vi "Collector.vi"(6 "MotorSpeed":dbl, 7 "Action":T10, 8 "Error in":errorcluster, 9 "BottomLS":T8={"DevStatus"={"status"=FALSE, "code"=0, "source"=""}, "DIO Channel"=enum."Invalid", "Digital Module"=enum."Digital Module 1"}, 10 "TopLS":T8={"DevStatus"={"status"=FALSE, "code"=0, "source"=""}, "DIO Channel"=enum."Invalid", "Digital Module"=enum."Digital Module 1"}, 11 "Motor":T1={"DeviceStatus"={"status"=FALSE, "code"=0, "source"=""}, "Type"=enum."PWM", "PWM"={"Digital Module"=enum."Digital Module 1", "PWM Channel"=enum."Invalid", "DeadBand"={"Name"="", "maxPositivePwm"=0, "minPositivePwm"=0, "centerPwm"=0, "maxNegativePwm"=0, "minNegativePwm"=0, "angularRange"=0}}, "CAN"={"Device Number"=0, "Control Mode"=enum."Percent VBus", "Semaphore"=refnum, "Max Vout"=12.0}, "Invert"=FALSE, "TransformRef"=refnum, "InvTransformRef"=refnum}) -> (0 "Error out":errorcluster, 1 "Lower Triggered?":bool, 2 "Upper Triggered?":bool)   [LabVIEW 2013]
doc: "Controls the collector arm, along with the two sets of limit switches associated with it (one set all the way up, the other all the way down). NOTE: all states return the status of the limit switches. It has the following actions:\n-Init: takes references to the motor and limit switches and stores them in shift registers\n-Raise: attempts to raise the collector (nothing happens if the upper limit switch is triggered)\n-Lower: attempts to lower the collector (nothing happens if the lower limit switch is triggered)\n-Stop: stops the motor\n-GetStatus: returns the value of the limit switches"
uses:
  CollectorAction.ctl
  <vilib>/Rock Robotics/WPI/DigitalInput/WPI_DigitalInputDevRef.ctl
  <vilib>/Rock Robotics/SystemInterfaces/DIO/FPGA_DIOChannel.ctl
  <vilib>/Rock Robotics/SystemInterfaces/Typedef/FPGA_TypedefDigitalModule.ctl
  <vilib>/Rock Robotics/WPI/MotorControl/WPI_MotorControlDeviceRef.ctl
  <vilib>/Rock Robotics/SystemInterfaces/DIO/FPGA_DIOPWMChannel.ctl
  <vilib>/Rock Robotics/WPI/PWM/WPI_PWMDeadband.ctl
  <vilib>/Rock Robotics/WPI/CAN/Jaguar/SubVIs/WPI_CANJaguar_ControlMode.ctl
  <vilib>/Rock Robotics/WPI/PWM/WPI_PWMTransform_ConPane.ctl
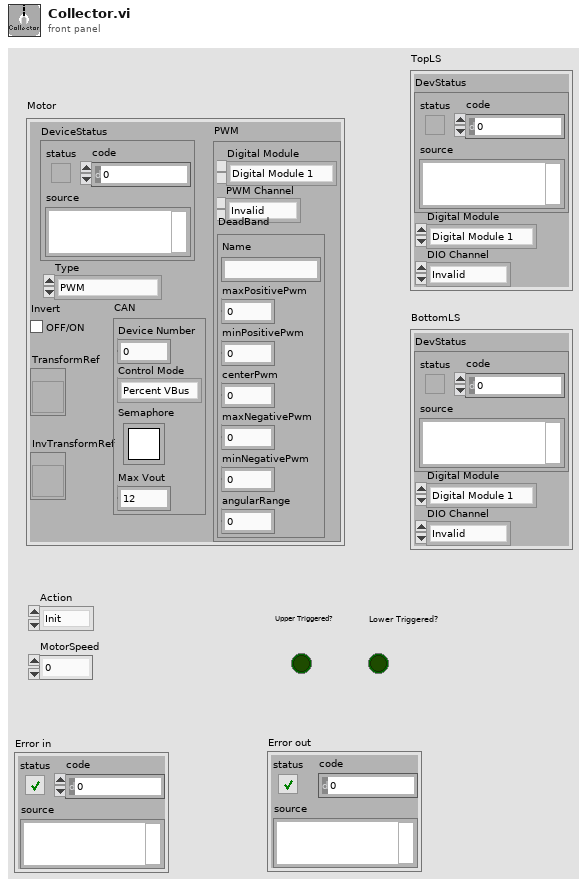
[diagram p1: front panel]
types:
  T1 = typedef "WPI_MotorControlDeviceRef.ctl" = cluster{"DeviceStatus":errorcluster, "Type":enum16{"PWM", "CAN"}, "PWM":cluster{"Digital Module":T2, "PWM Channel":T3, "DeadBand":T4}, "CAN":cluster{"Device Number":u8, "Control Mode":T5, "Semaphore":T6, "Max Vout":dbl}, "Invert":bool, "TransformRef":T7, "InvTransformRef":T7}
  T2 = typedef "FPGA_TypedefDigitalModule.ctl" = enum16{"Digital Module 1", "Digital Module 2"}
  T3 = typedef "FPGA_DIOPWMChannel.ctl" = enum8{"PWM 1", "PWM 2", "PWM 3", "PWM 4", "PWM 5", "PWM 6", "PWM 7", "PWM 8", "PWM 9", "PWM 10", "Invalid"}
  T4 = typedef "WPI_PWMDeadband.ctl" = cluster{"Name":string, "maxPositivePwm":i32, "minPositivePwm":i32, "centerPwm":i32, "maxNegativePwm":i32, "minNegativePwm":i32, "angularRange":u16}
  T5 = typedef "WPI_CANJaguar_ControlMode.ctl" = enum8{"Percent VBus", "Current", "Speed", "Position", "Voltage"}
  T6 = typedef "Semaphore RefNum" = refnum<k1>
  T7 = typedef "WPI_PWMTransform_ConPane.ctl" = refnum<vi>
  T8 = typedef "WPI_DigitalInputDevRef.ctl" = cluster{"DevStatus":errorcluster, "DIO Channel":T9, "Digital Module":T2}
  T9 = typedef "FPGA_DIOChannel.ctl" = enum8{"DIO 1", "DIO 2", "DIO 3", "DIO 4", "DIO 5", "DIO 6", "DIO 7", "DIO 8", "DIO 9", "DIO 10", "DIO 11", "DIO 12", "DIO 13", "DIO 14", "Invalid"}
  T10 = typedef "CollectorAction.ctl" = enum16{"Init", "Raise", "Lower", "Stop", "GetStatus"}
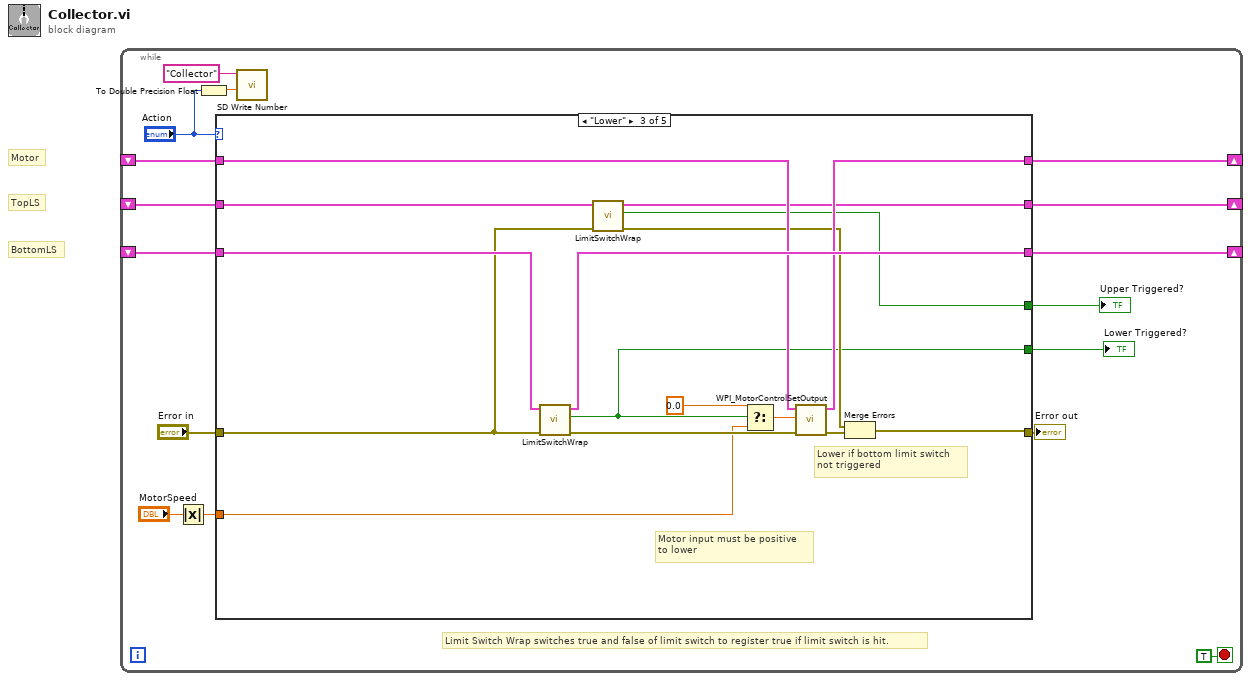
[diagram p0: block diagram]
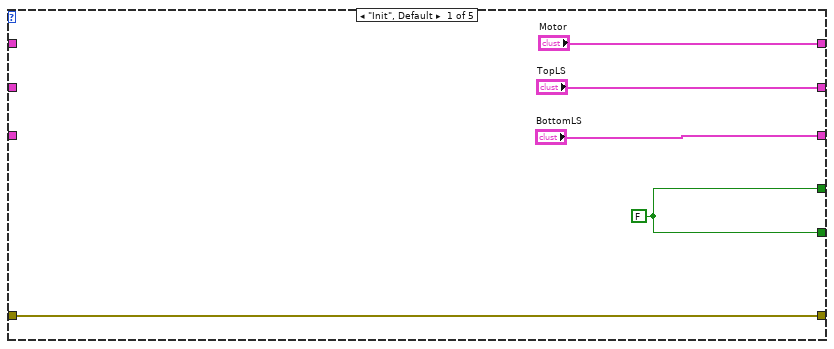
[diagram p2: hidden frame]
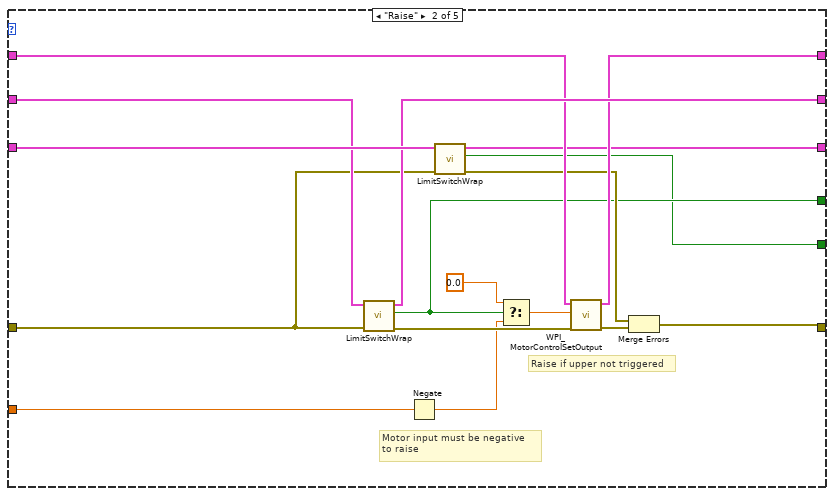
[diagram p3: hidden frame]
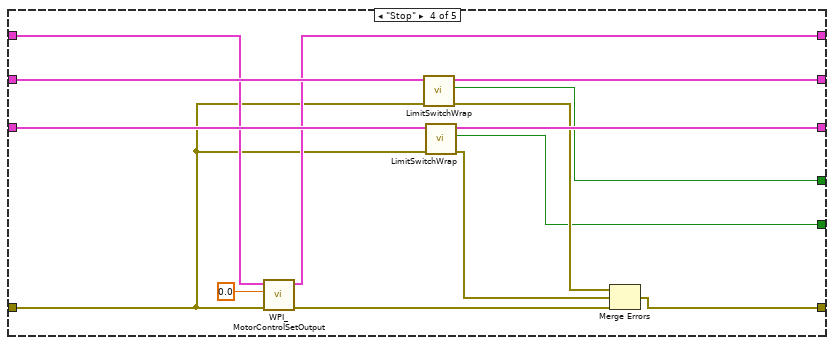
[diagram p4: hidden frame]
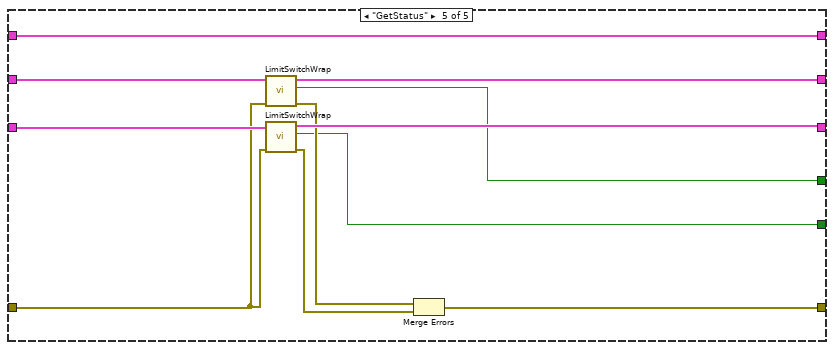
[diagram p5: hidden frame]
diagram:
  # "BottomLS"
  # "TopLS"
  # "Motor"
  n1 = while {
    shift-right: [w13] -> _
    shift-left: _ -> [w10]
    shift-right: [w14] -> _
    shift-left: _ -> [w11]
    shift-right: [w15] -> _
    shift-left: _ -> [w12]
    stop <- TRUE stop-if-true
    # "Limit Switch Wrap switches true and false of limit switch to register true if limit switch is hit."
    n2 = Absolute Value(x="MotorSpeed") -> (abs(x)=w4:dbl)
    n3 = To Double Precision Float(number="Action") -> (double precision float=w1:dbl)
    n4 = case shown="\"Lower\"" "Action" {
      tunnel: ["Motor" w31 w47 w64 w79] -> w15
      tunnel: ["TopLS" w33 w46 w62 w76] -> w14
      tunnel: ["BottomLS" w30 w50 w63 w75] -> w13
      tunnel: w12 -> [_ w32 w48 w65 w79]
      tunnel: w11 -> [_ w34 w54 w67 w77]
      tunnel: w10 -> [_ w38 w51 w66 w78]
      tunnel: "Error in" -> [w21 w29 w45 w61 w74]
      tunnel: [w21 w27 w44 w59 w71] -> w8
      tunnel: [w17 w24 w40 w56 w70] -> w6
      tunnel: [w17 w25 w41 w55 w69] -> w7
      tunnel: w4 -> [_ w23 w39 _ _]
      frame "Init", Default {
        w17 = FALSE
      }
      frame "Raise" {
        # "Motor input must be negative\nto raise"
        # "Raise if upper not triggered"
        n5 = call "LimitSwitchWrap.vi"("error in"=w29, "DigitalInputDevRef"=w34) -> ("error out"=w35:errorcluster, "Triggered"=w25:bool, "DigitalInputDevRef 2"=w33:T8)  [unwired: 7 in]
        n6 = Negate(x=w23) -> (-x=w22:dbl)
        n7 = call "LimitSwitchWrap.vi"("error in"=w29, "DigitalInputDevRef"=w38) -> ("error out"=w26:errorcluster, "Triggered"=w24:bool, "DigitalInputDevRef 2"=w30:T8)  [unwired: 7 in]
        n8 = Select(t=0.0, s=w25, f=w22) -> (s? t:f=w37:dbl)
        n9 = call <vilib>:"WPI_MotorControlSetOutput.vi"("error in (no error)"=w35, "Output"=w37, "MotorControlDevRef"=w32) -> ("error out"=w28:errorcluster, "MotorControlDevRef"=w31:T1)  [unwired: 6 in, 1 out]
        n10 = Merge Errors(w26, w28) -> (w27:errorcluster)
      }
      frame "Lower" {
        # "Motor input must be positive\nto lower"
        # "Lower if bottom limit switch\nnot triggered"
        n11 = call "LimitSwitchWrap.vi"("error in"=w45, "DigitalInputDevRef"=w51) -> ("error out"=w49:errorcluster, "Triggered"=w40:bool, "DigitalInputDevRef 2"=w50:T8)  [unwired: 7 in]
        n12 = call "LimitSwitchWrap.vi"("error in"=w45, "DigitalInputDevRef"=w54) -> ("error out"=w42:errorcluster, "Triggered"=w41:bool, "DigitalInputDevRef 2"=w46:T8)  [unwired: 7 in]
        n13 = Select(t=0.0, s=w40, f=w39) -> (s? t:f=w53:dbl)
        n14 = call <vilib>:"WPI_MotorControlSetOutput.vi"("error in (no error)"=w49, "Output"=w53, "MotorControlDevRef"=w48) -> ("error out"=w43:errorcluster, "MotorControlDevRef"=w47:T1)  [unwired: 6 in, 1 out]
        n15 = Merge Errors(w42, w43) -> (w44:errorcluster)
      }
      frame "Stop" {
        n16 = call <vilib>:"WPI_MotorControlSetOutput.vi"("error in (no error)"=w61, "Output"=0.0, "MotorControlDevRef"=w65) -> ("error out"=w60:errorcluster, "MotorControlDevRef"=w64:T1)  [unwired: 6 in, 1 out]
        n17 = call "LimitSwitchWrap.vi"("error in"=w61, "DigitalInputDevRef"=w67) -> ("error out"=w57:errorcluster, "Triggered"=w55:bool, "DigitalInputDevRef 2"=w62:T8)  [unwired: 7 in]
        n18 = call "LimitSwitchWrap.vi"("error in"=w61, "DigitalInputDevRef"=w66) -> ("error out"=w58:errorcluster, "Triggered"=w56:bool, "DigitalInputDevRef 2"=w63:T8)  [unwired: 7 in]
        n19 = Merge Errors(w57, w58, w60) -> (w59:errorcluster)
      }
      frame "GetStatus" {
        n20 = call "LimitSwitchWrap.vi"("error in"=w74, "DigitalInputDevRef"=w77) -> ("error out"=w72:errorcluster, "Triggered"=w69:bool, "DigitalInputDevRef 2"=w76:T8)  [unwired: 7 in]
        n21 = call "LimitSwitchWrap.vi"("error in"=w74, "DigitalInputDevRef"=w78) -> ("error out"=w73:errorcluster, "Triggered"=w70:bool, "DigitalInputDevRef 2"=w75:T8)  [unwired: 7 in]
        n22 = Merge Errors(w72, w73) -> (w71:errorcluster)
      }
    }
    "Error out" <- w8
    "Upper Triggered?" <- w7
    "Lower Triggered?" <- w6
    n23 = call <vilib>:"SD Write Number.vi"("Numeric"=w1, "Name"="Collector") -> ()  [unwired: 8 in, 2 out]
  }
